vi "ma_FFT Spectrum no State.vi"(0 "time signal":waveform(dbl), 1 "restart averaging (F)":bool, 2 "mag-phase":bool, 5 "window":T3=1 items=["Rectangle"=0, "Hanning"=1, "Hamming"=2, "Blackman-Harris"=3, "Exact Blackman"=4, "Blackman"=5, "Flat Top"=6, "4 Term B-Harris "=7, "7 Term B-Harris"=8, "Low Sidelobe"=9, "Blackman Nuttall"=11, "Triangle"=30, "Bartlett-Hanning"=31, "Bohman"=32, "Parzen"=33, "Welch"=34, "Kaiser"=60, "Dolph-Chebyshev"=61, "Gaussian"=62], 7 "averaging parameters":T5={"averaging mode"=enum."No averaging", "weighting mode"=enum."Exponential", "number of averages"=10} {"number of averages" min=1}, 9 "view":T2, 11 "error in":errorcluster, 12 "state info":T4 {"real spectrum" format="%0.2f"; "averages completed" format="%0.2f"; "df" format="%0.2f"; "complex spectrum" format="%0.2f"; "spectrum parameters"."window" items=["Rectangle"=0, "Hanning"=1, "Hamming"=2, "Blackman-Harris"=3, "Exact Blackman"=4, "Blackman"=5, "Flat Top"=6, "4 Term B-Harris "=7, "7 Term B-Harris"=8, "Low Sidelobe"=9, "Blackman Nuttall"=11, "Triangle"=30, "Bartlett-Hanning"=31, "Bohman"=32, "Parzen"=33, "Welch"=34, "Kaiser"=60, "Dolph-Chebyshev"=61, "Gaussian"=62]; "dt" format="%0.2f"; "timestamp" format="%0.2f"; "dt history" format="%0.2f"; "t0 history" format="%0.2f"}, 13 "window parameter":dbl=nan) -> (3 "averaging done":bool, 4 "real or mag":cluster{"f0":dbl, "df":dbl, "real or mag":dbl[]} {"f0" format="%0.2p"; "df" format="%0.2p"; "real or mag" format="%0.2p"}, 6 "imag or phase":T1 {"f0" format="%0.2p"; "df" format="%0.2p"; "imag or phase" format="%0.2p"}, 10 "averages completed":dbl format="%0.2f", 14 "state info":T4 {"real spectrum" format="%0.2f"; "averages completed" format="%0.2f"; "df" format="%0.2f"; "complex spectrum" format="%0.2f"; "spectrum parameters"."window" items=["Rectangle"=0, "Hanning"=1, "Hamming"=2, "Blackman-Harris"=3, "Exact Blackman"=4, "Blackman"=5, "Flat Top"=6, "4 Term B-Harris "=7, "7 Term B-Harris"=8, "Low Sidelobe"=9, "Blackman Nuttall"=11, "Triangle"=30, "Bartlett-Hanning"=31, "Bohman"=32, "Parzen"=33, "Welch"=34, "Kaiser"=60, "Dolph-Chebyshev"=61, "Gaussian"=62]; "dt" format="%0.2f"; "timestamp" format="%0.2f"; "dt history" format="%0.2f"; "t0 history" format="%0.2f"}, 15 "error out":errorcluster)   [LabVIEW 2020, in "NI_MAPro.lvlib"]
doc: "Computes the averaged auto power spectrum of the input signal. Each time waveform corresponds to a single FFT block and has to be passed individually to this VI. Averaging parameters specifies how the averaging is performed. This includes the averaging mode (No averaging, vector averaging, RMS averaging, or peak hold), the weighting mode (linear or exponential), and the number of averages. Averages completed returns the number of averages completed so far."
uses:
  NI_MAPro.lvlib
  windowTd.ctl
  NI_AALPro.lvlib
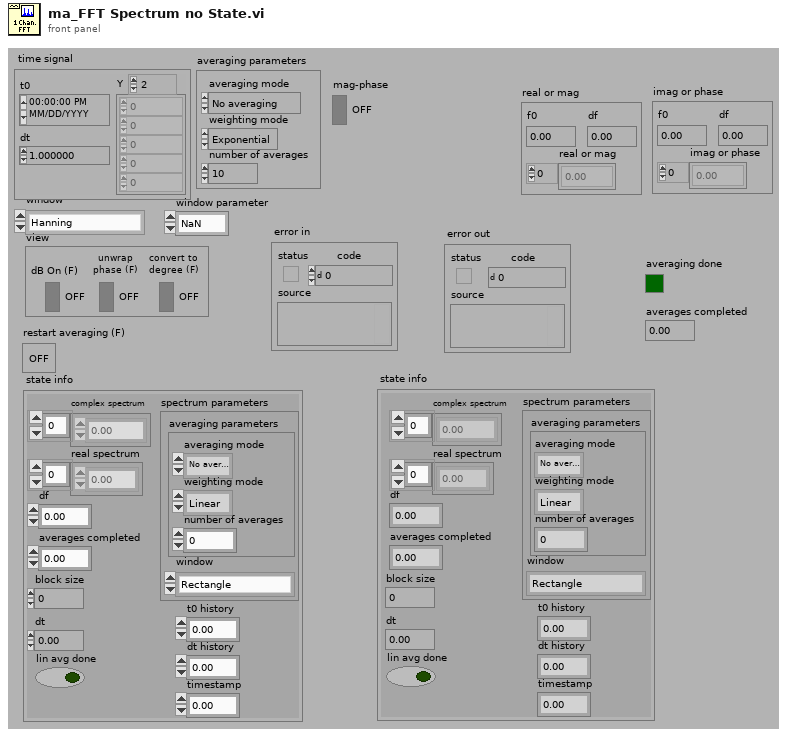
[diagram p1: front panel]
types:
  T1 = cluster{"f0":dbl, "df":dbl, "imag or phase":dbl[]}
  T2 = cluster{"dB On (F)":bool, "unwrap phase (F)":bool, "convert to degree (F)":bool}
  T3 = typedef "NI_AALPro.lvlib/windowTd.ctl" = u32
  T4 = cluster{"block size":i32, "dt":dbl, "spectrum parameters":cluster{"averaging parameters":cluster{"averaging mode":enum16{"No averaging", "Vector averaging", "RMS averaging", "Peak hold"}, "weighting mode":enum16{"Linear", "Exponential"}, "number of averages":u32}, "window":T3}, "df":dbl, "averages completed":dbl, "complex spectrum":cdb[], "real spectrum":dbl[], "t0 history":dbl, "dt history":dbl, "timestamp":dbl, "lin avg done":bool}
  T5 = cluster{"averaging mode":enum16{"No averaging", "Vector averaging", "RMS averaging", "Peak hold"}, "weighting mode":enum16{"Linear", "Exponential"}, "number of averages":u32}
  T6 = enum16{"FFT spectrum", "Power spectrum", "Cross spectrum", "Frequency response"}
  T7 = enum16{"No averaging", "Vector averaging", "RMS averaging", "Peak hold"}
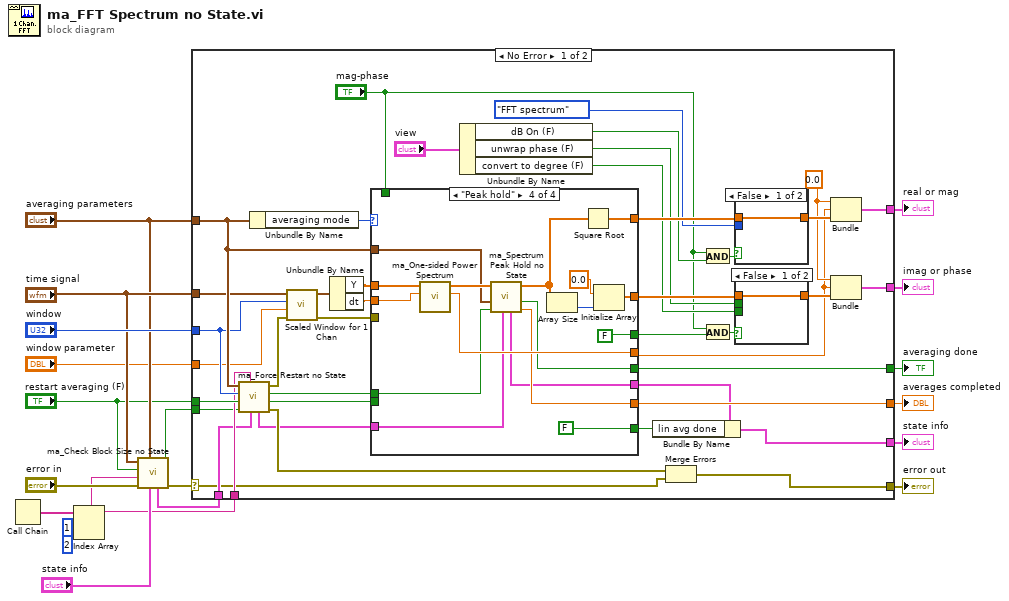
[diagram p0: block diagram]
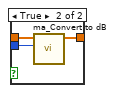
[diagram p2: hidden frame]
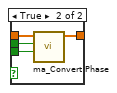
[diagram p3: hidden frame]
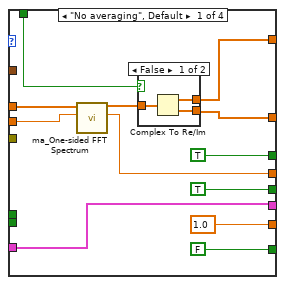
[diagram p4: hidden frame]
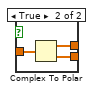
[diagram p5: hidden frame]
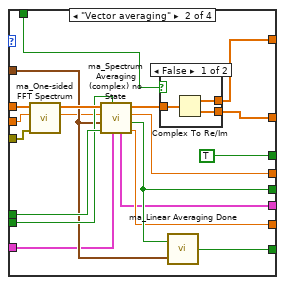
[diagram p6: hidden frame]
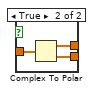
[diagram p7: hidden frame]
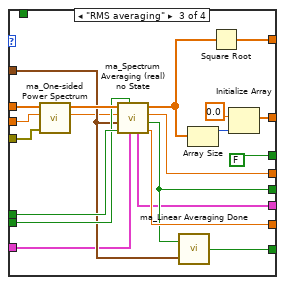
[diagram p8: hidden frame]
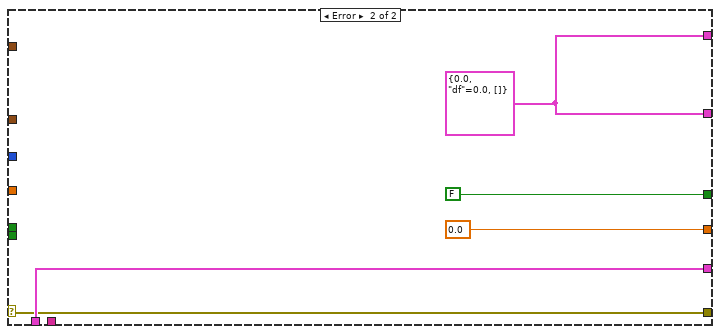
[diagram p9: hidden frame]
diagram:
  n1 = Call Chain() -> (call chain=w6:string[])
  n2 = Index Array(array=w6, index #1=1 ("Index"), index #2=2 ("Index")) -> (element #1=w5:string)  [unwired: 1 out]
  n3 = call "ma_Check Block Size no State.vi"("state info"="state info", "averaging parameters"="averaging parameters", "error in"="error in", "caller VI name"=w5, "restart averaging (F)"="restart averaging (F)", "time signal"="time signal") -> ("error out"=w14:errorcluster, "force restart averaging"=w3:bool, "state info"=w10:T4)  [unwired: 3 out]
  n4 = case shown="No Error" w14 {
    selector: w14 -> [w22 w152]
    tunnel: "averaging parameters" -> [w62 _]
    tunnel: [w61 0.0] -> w20
    tunnel: "window" -> [w60 _]
    tunnel: [w59 FALSE ("averaging done")] -> w18
    tunnel: "time signal" -> [w58 _]
    tunnel: "restart averaging (F)" -> [w57 _]
    tunnel: [w55 w152] -> w16
    tunnel: [w28 w153] -> w12
    tunnel: w5 -> [w54 _]
    tunnel: w10 -> [w42 w154]
    tunnel: [w52 w154] -> w9
    tunnel: [w29 w153] -> w4
    tunnel: w3 -> [w23 _]
    tunnel: "window parameter" -> [w21 _]
    frame No Error {
      w37 = 0.0
      n5 = call "ma_Force Restart no State.vi"("state info"=w42, "caller VI name"=w54, "force restart averaging in"=w23, "restart averaging (F)"=w57, "window"=w60, "averaging parameters"=w62) -> ("error out"=w56:errorcluster, "retrieve last spectrum"=w44:bool, "force restart averaging"=w45:bool, "skip processing"=w46:errorcluster, "state info"=w43:T4)  [unwired: 1 out]
      n6 = Unbundle By Name(w62) -> ("averaging mode"=w51:T7)
      n7 = call "Scaled Window for 1 Chan.vi"("error in (no error)"=w46, "window parameter"=w21, "window"=w60, "signal in"=w58) -> ("error out"=w50:errorcluster, "signal out"=w47:waveform(dbl))  [unwired: 5 in, 1 out]
      n8 = Unbundle By Name(w47) -> ("Y"=w48:dbl[], "dt"=w49:dbl)
      n9 = case shown="\"Peak hold\"" w51 {
        tunnel: w48 -> [w79 w106 w133 w151]
        tunnel: [w76 w93 w126 w149] -> w30
        tunnel: [w75 w91 w120 w140] -> w36
        tunnel: w62 -> [_ w100 w127 w143]
        tunnel: w45 -> [_ w108 w134 w147]
        tunnel: [1.0 ("averages completed") w97 w124 w146] -> w61
        tunnel: w49 -> [w78 w105 w132 w150]
        tunnel: [TRUE ("averaging done") w98 w123 w144] -> w59
        tunnel: [FALSE w103 w130 FALSE] -> w53
        tunnel: w50 -> [_ w102 w129 _]
        tunnel: w44 -> [_ w101 w128 _]
        tunnel: w43 -> [w80 w96 w122 w142]
        tunnel: [w80 w95 w121 w141] -> w41
        tunnel: [w74 w92 w116 w136] -> w35
        tunnel: [TRUE ("averaging done") TRUE FALSE FALSE] -> w31
        tunnel: "mag-phase" -> [w72 w90 _ _]
        frame "No averaging", Default {
          n10 = call "ma_One-sided FFT Spectrum.vi"("dt"=w78, "signal (V)"=w79) -> ("df"=w76:dbl, "FFT spectrum (Vrms)"=w73:cdb[])  [unwired: 1 in, 7 out]
          n11 = case shown="False" w72 {
            tunnel: w73 -> [w86 w89]
            tunnel: [w85 w88] -> w75
            tunnel: [w84 w87] -> w74
            frame False {
              n12 = Complex To Re/Im(x + iy=w86) -> (x=w85:dbl[], y=w84:dbl[])
            }
            frame True {
              n13 = Complex To Polar(r * e^(i*theta)=w89) -> (r=w88:dbl[], theta=w87:dbl[])
            }
          }
        }
        frame "Vector averaging" {
          n14 = call "ma_One-sided FFT Spectrum.vi"("error in"=w102, "dt"=w105, "signal (V)"=w106) -> ("df"=w99:dbl, "FFT spectrum (Vrms)"=w104:cdb[])  [unwired: 7 out]
          n15 = call "ma_Spectrum Averaging (complex) no State.vi"("state info"=w96, "retrieve last spectrum (F)"=w101, "restart averaging (F)"=w108, "averaging parameters"=w100, "df"=w99, "complex spectrum"=w104) -> ("averages completed"=w97:dbl, "averaging done"=w98:bool, "df"=w93:dbl, "averaged complex spectrum"=w107:cdb[], "state info"=w95:T4)  [unwired: 1 out]
          n16 = case shown="False" w90 {
            tunnel: w107 -> [w111 w114]
            tunnel: [w110 w113] -> w91
            tunnel: [w109 w112] -> w92
            frame False {
              n17 = Complex To Re/Im(x + iy=w111) -> (x=w110:dbl[], y=w109:dbl[])
            }
            frame True {
              n18 = Complex To Polar(r * e^(i*theta)=w114) -> (r=w113:dbl[], theta=w112:dbl[])
            }
          }
          n19 = call "ma_Linear Averaging Done.vi"("averaging parameters"=w100, "averaging done"=w98) -> ("linear averaging done"=w103:bool)
        }
        frame "RMS averaging" {
          n20 = call "ma_One-sided Power Spectrum.vi"("error in"=w129, "dt"=w132, "signal (V)"=w133) -> ("df"=w125:dbl, "power spectrum (V^2 rms)"=w131:dbl[])  [unwired: 7 out]
          n21 = call "ma_Spectrum Averaging (real) no State.vi"("state info"=w122, "retrieve last spectrum (F)"=w128, "restart averaging (F)"=w134, "averaging parameters"=w127, "df"=w125, "real spectrum"=w131) -> ("averages completed"=w124:dbl, "averaging done"=w123:bool, "df"=w126:dbl, "averaged real spectrum"=w117:dbl[], "state info"=w121:T4)  [unwired: 1 out]
          n22 = call "ma_Linear Averaging Done.vi"("averaging parameters"=w127, "averaging done"=w123) -> ("linear averaging done"=w130:bool)
          n23 = Array Size(array=w117) -> (size(s)=w118:i32)
          n24 = Square Root(x=w117) -> (sqrt(x)=w120:dbl[])
          n25 = Initialize Array(0.0, w118) -> (w116:dbl[])
        }
        frame "Peak hold" {
          n26 = call "ma_One-sided Power Spectrum.vi"("dt"=w150, "signal (V)"=w151) -> ("df"=w149:dbl, "power spectrum (V^2 rms)"=w148:dbl[])  [unwired: 1 in, 7 out]
          n27 = call "ma_Spectrum Peak Hold no State.vi"("state info"=w142, "restart averaging (F)"=w147, "averaging parameters"=w143, "real spectrum"=w148) -> ("averages completed"=w146:dbl, "averaging done"=w144:bool, "peak spectrum"=w137:dbl[], "state info"=w141:T4)  [unwired: 4 out]
          n28 = Array Size(array=w137) -> (size(s)=w138:i32)
          n29 = Square Root(x=w137) -> (sqrt(x)=w140:dbl[])
          n30 = Initialize Array(0.0, w138) -> (w136:dbl[])
        }
      }
      n31 = Unbundle By Name("view") -> ("dB On (F)"=w33:bool, "unwrap phase (F)"=w27:bool, "convert to degree (F)"=w26:bool)
      n32 = Bundle By Name(cluster=w41, "lin avg done"=w53) -> (w52:T4)
      n33 = Merge Errors(w56, w22) -> (w55:errorcluster)
      n34 = And(x="mag-phase", y=w33) -> (x .and. y?=w34:bool)
      n35 = And(x="mag-phase", y=w31) -> (x .and. y?=w32:bool)
      n36 = case shown="False" w34 {
        tunnel: [w63 w65] -> w39
        tunnel: w36 -> [w63 w66]
        tunnel: T6."FFT spectrum" ("spectrum type") -> [_ w64]
        frame False {
        }
        frame True {
          n37 = call "ma_Convert to dB.vi"("spectrum type"=w64, "spectrum"=w66) -> ("spectrum in dB"=w65:dbl[])  [unwired: 9 out]
        }
      }
      n38 = case shown="False" w32 {
        tunnel: [w67 w68] -> w38
        tunnel: w35 -> [w67 w71]
        tunnel: w27 -> [_ w70]
        tunnel: w26 -> [_ w69]
        frame False {
        }
        frame True {
          n39 = call "ma_Convert Phase.vi"("convert to degree (F)"=w69, "unwrap phase (F)"=w70, "phase (radian)"=w71) -> ("scaled phase"=w68:dbl[])  [unwired: 3 in, 5 out]
        }
      }
      n40 = Bundle(w37, "df"=w30, "spectrum in dB"=w39) -> (w28:cluster{dbl, "df":dbl, "spectrum in dB":dbl[]})  [unwired: 1 out]
      n41 = Bundle(w37, "df"=w30, "scaled phase"=w38) -> (w29:cluster{dbl, "df":dbl, "scaled phase":dbl[]})  [unwired: 1 out]
    }
    frame Error {
      w153 = cluster{dbl, "df":dbl, dbl[]} {0.0, "df"=0.0, []}
    }
  }
  "averages completed" <- w20
  "error out" <- w16
  "averaging done" <- w18
  "real or mag" <- w12
  "state info" <- w9
  "imag or phase" <- w4
